vi "Serialized Device Cfg FG.vi"(7 "State":enum16{"Add Entry", "Init", "Get"}(ring)=enum."Get", 11 "CfgStrIn":string) -> (3 "SerializedStrOut":string)   [LabVIEW 2014, in "DAQ Device.lvlib"]
uses:
  reusable/DAQ Device/DAQ Device.lvlib
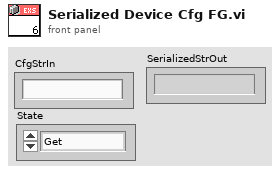
[diagram p1: front panel]
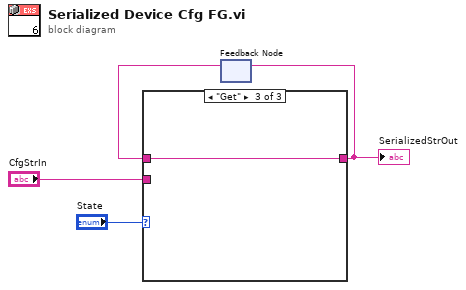
[diagram p0: block diagram]
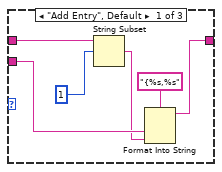
[diagram p2: hidden frame]
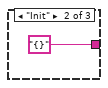
[diagram p3: hidden frame]
diagram:
  n1 = feedback #1() -> (w1:string)  [unwired: 1 in]
  n2 = case shown="\"Get\"" "State" {
    tunnel: "CfgStrIn" -> [w7 _ _]
    tunnel: [w5 "{}" w12] -> w2
    tunnel: w1 -> [w10 _ w12]
    frame "Add Entry", Default {
      n3 = String Subset(string=w10, offset (0)=1) -> (substring=w6:string)  [unwired: 1 in]
      n4 = Format Into String(format string="{%s,%s", w7, w6) -> (resulting string=w5:string)  [unwired: 2 in, 1 out]
    }
    frame "Init" {
    }
    frame "Get" {
    }
  }
  "SerializedStrOut" <- w2
  n5 = feedback-in #1(w2) -> ()
